vi "Resource Check.vi"() -> (4 "C: free (GB)":dbl, 6 "D: free (GB)":dbl, 8 "Free memory (%)":dbl, 15 "error out":errorcluster)   [LabVIEW 2010]
uses:
  kernel32.dll
panel:
  out "Available":dbl
  out "Total":dbl
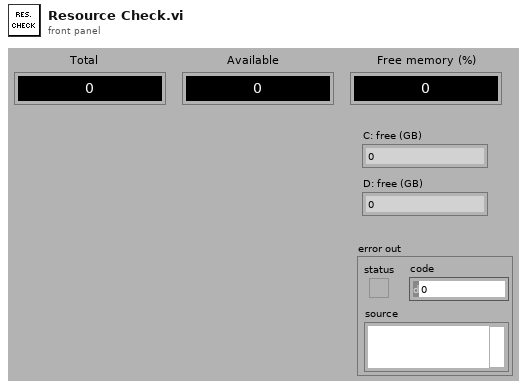
[diagram p1: front panel]
types:
  T1 = cluster{"dwLength":u32, "dwMemoryLoad":u32, "ullTotalPhys":u64, "ullAvailPhys":u64, "ullTotalPageFile":u64, "ullAvailPageFile":u64, "ullTotalVirtual":u64, "ullAvailVirtual":u64, "ullAvailExtendedVirtual":u64}
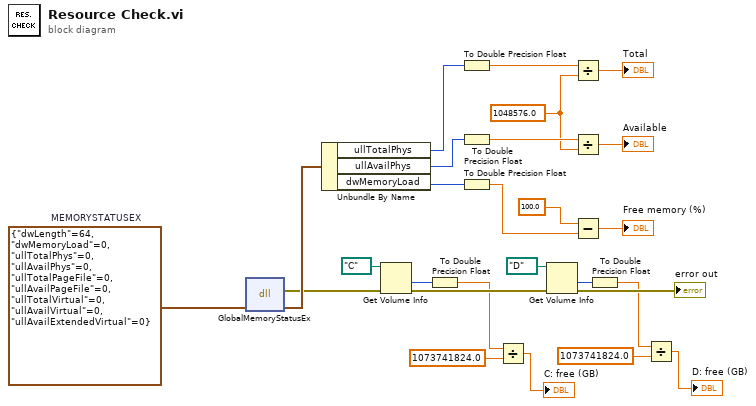
[diagram p0: block diagram]
diagram:
  w12 = 1048576.0 ("y")
  w17 = T1 {"dwLength"=64, "dwMemoryLoad"=0, "ullTotalPhys"=0, "ullAvailPhys"=0, "ullTotalPageFile"=0, "ullAvailPageFile"=0, "ullTotalVirtual"=0, "ullAvailVirtual"=0, "ullAvailExtendedVirtual"=0}  # MEMORYSTATUSEX
  n1 = dll-call lib="kernel32.dll" fn="GlobalMemoryStatusEx"(w17) -> (error out=w4:errorcluster, w11:T1)  [unwired: 4 in, 1 out]
  n2 = Unbundle By Name(w11) -> ("ullTotalPhys"=w16:u64, "ullAvailPhys"=w14:u64, "dwMemoryLoad"=w8:u32)
  n3 = Get Volume Info(8:w4, 11:path "C:/" ("path")) -> (0:w24:errorcluster, 1:w22:i64)  [unwired: 4 out]
  n4 = To Double Precision Float(number=w22) -> (double precision float=w2:dbl)
  n5 = To Double Precision Float(number=w16) -> (double precision float=w15:dbl)
  n6 = To Double Precision Float(number=w14) -> (double precision float=w13:dbl)
  n7 = To Double Precision Float(number=w8) -> (double precision float=w6:dbl)
  n8 = Divide(x=w2, y=1073741824.0) -> (x/y=→"C: free (GB)":dbl)
  n9 = Get Volume Info(8:w24, 11:path "D:/" ("path")) -> (0:→"error out":errorcluster, 1:w3:i64)  [unwired: 4 out]
  n10 = Divide(x=w15, y=w12) -> (x/y=→"Total":dbl)
  n11 = Divide(x=w13, y=w12) -> (x/y=→"Available":dbl)
  n12 = Subtract(x=100.0, y=w6) -> (x-y=→"Free memory (%)":dbl)
  n13 = To Double Precision Float(number=w3) -> (double precision float=w1:dbl)
  n14 = Divide(x=w1, y=1073741824.0) -> (x/y=→"D: free (GB)":dbl)
